vi "仪器参数改变发送 (子VI).vi"(8 "错误输入":errorcluster caption="错误输出") -> (0 "错误输出":errorcluster)   [LabVIEW 2016, in "数据传输系统-06.lvlib"]
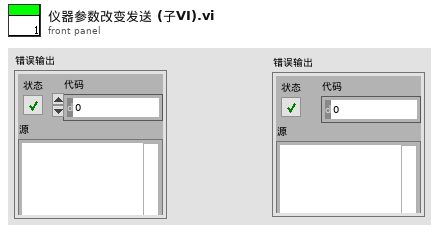
[diagram p1: front panel]
types:
  T1 = cluster{"测量量程":dbl, "测量精度":dbl, "测量间隔":dbl, "消解温度":dbl, "消解时长":dbl, "空白校准时间":timestamp, "曲线截距":dbl, "曲线斜率":dbl, "测量检出限":dbl, "测量信号值":dbl, "线性相关系数":dbl, "二次多项式系数":dbl, "标样校准时间":timestamp, "稀释倍数":dbl, "三项式系数":dbl, "空白标定系数":dbl, "量程系数":dbl, "F0/ORPA":dbl, "F1/ORPB":dbl, "F2/ORPK":dbl, "F3":dbl, "F4":dbl, "F5":dbl, "F6":dbl, "F7":dbl, "X0/滴定数":dbl, "量程":dbl}
  T2 = cluster{"CODMn关键参数":bool, "氨氮关键参数":bool, "总磷关键参数":bool, "总氮关键参数":bool, "CODCr关键参数":bool, "采配水关键参数":bool}
  T3 = cluster{"测量量程":dbl, "测量精度":dbl, "测量间隔":dbl, "消解温度":dbl, "消解时长":dbl, "空白校准时间":timestamp, "曲线截距":dbl, "曲线斜率":dbl, "测量检出限":dbl, "测量信号值":dbl, "线性相关系数":dbl, "二次多项式系数":dbl, "标样校准时间":timestamp, "稀释倍数":dbl, "三项式系数":dbl, "空白标定系数":dbl, "量程系数":dbl, "F0/ORPA":dbl, "F1/ORPB":dbl, "F2/ORPK":dbl, "F3":dbl, "F4":dbl, "F5":dbl, "F6":dbl, "F7":dbl, "X0/滴定数":dbl, "量程":dbl}[]
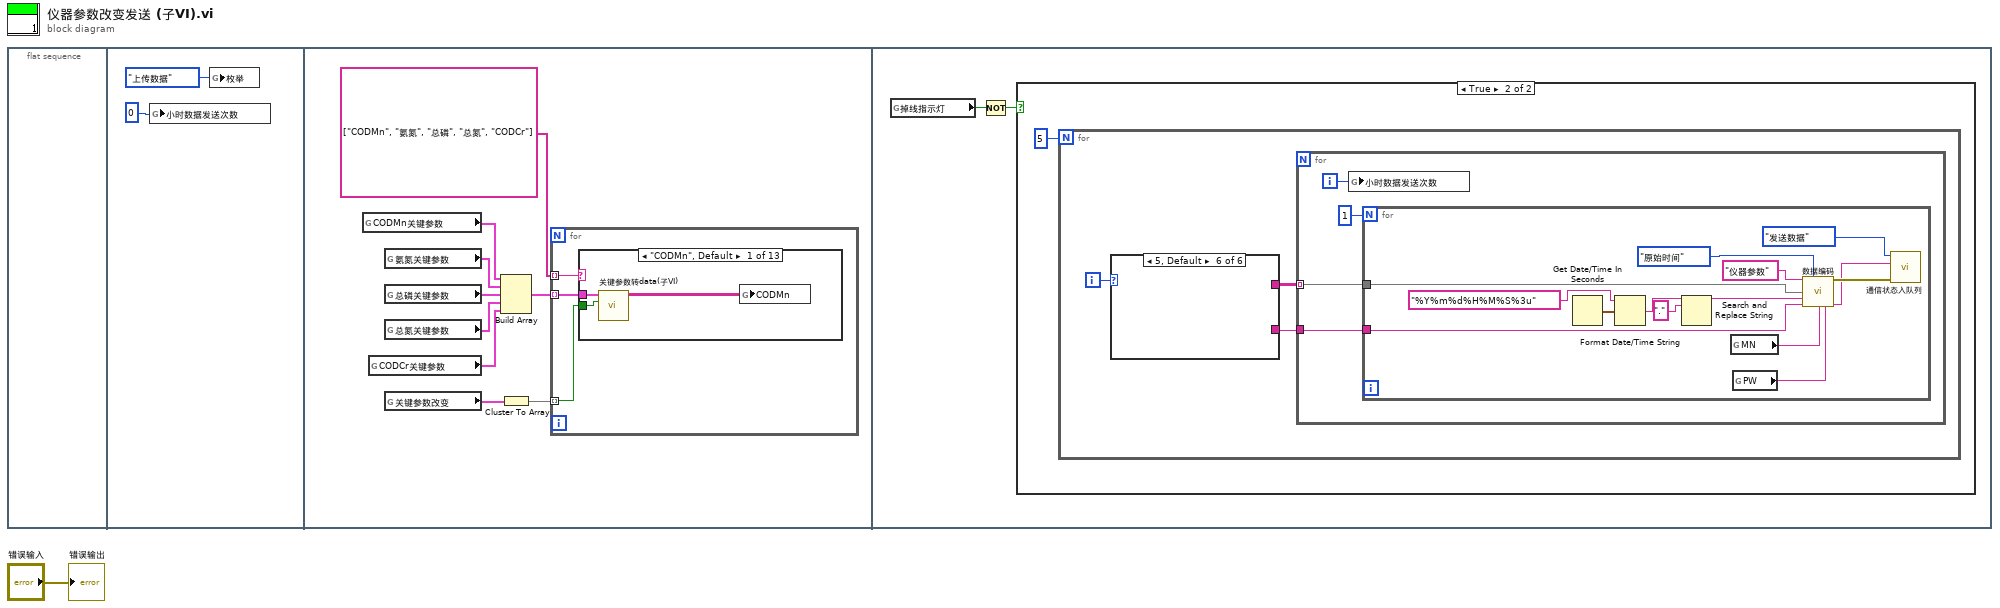
[diagram p0: block diagram]
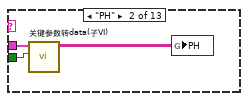
[diagram p2: hidden frame]
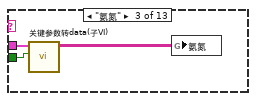
[diagram p3: hidden frame]
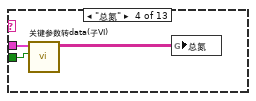
[diagram p4: hidden frame]
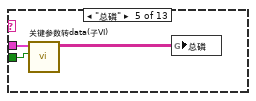
[diagram p5: hidden frame]
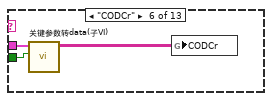
[diagram p6: hidden frame]
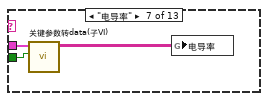
[diagram p7: hidden frame]
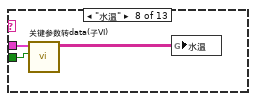
[diagram p8: hidden frame]
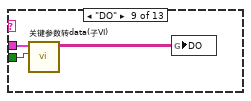
[diagram p9: hidden frame]
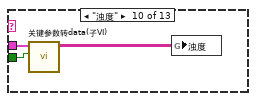
[diagram p10: hidden frame]
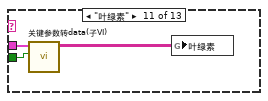
[diagram p11: hidden frame]
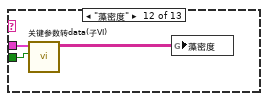
[diagram p12: hidden frame]
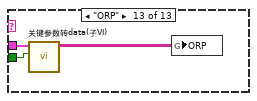
[diagram p13: hidden frame]
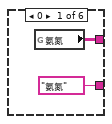
[diagram p15: hidden frame]
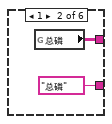
[diagram p16: hidden frame]
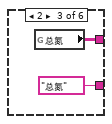
[diagram p17: hidden frame]
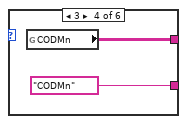
[diagram p18: hidden frame]
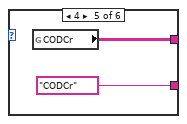
[diagram p19: hidden frame]
diagram:
  n1 = flat-sequence {
    frame #0 {
    }
    frame #1 {
      n2 = global write "全局 小时数据发送次数.vi" "小时数据发送次数"(0 ("小时数据发送次数")) -> ()
      n3 = global write "全局1.vi" "枚举"(enum16{"返回请求应答", "上传数据", "返回执行结果"}."上传数据" ("枚举")) -> ()
    }
    frame #2 {
      n4 = global read "全局1.vi" "CODMn关键参数"() -> (w9:T1)
      n5 = global read "全局1.vi" "CODCr关键参数"() -> (w12:T1)
      n6 = global read "全局1.vi" "氨氮关键参数"() -> (w11:T1)
      n7 = global read "全局1.vi" "总磷关键参数"() -> (w7:T1)
      n8 = global read "全局1.vi" "总氮关键参数"() -> (w6:T1)
      n9 = global read "全局1.vi" "关键参数改变"() -> (w5:T2)
      n10 = Build Array(w9, w11, w7, w6, w12) -> (w10:T3)
      n11 = Cluster To Array(cluster=w5) -> (array=w4:bool[])
      n12 = for {
        tunnel: string[] ["CODMn", "氨氮", "总磷", "总氮", "CODCr"] -> [w15] mode=indexing
        tunnel: w10 -> [w14] mode=indexing
        tunnel: w4 -> [w13] mode=indexing
        n13 = case shown="\"CODMn\", Default" w15 {
          tunnel: w14 -> [w17 w21 w24 w27 w30 w33 w36 w39 w42 w45 w48 w51 w54]
          tunnel: w13 -> [w16 w19 w22 w25 w28 w31 w34 w37 w40 w43 w46 w49 w52]
          frame "CODMn", Default {
            n14 = call "关键参数转data(子VI).vi"("改变?"=w16, "关键参数"=w17) -> ("数组"=w18:string[][])  [unwired: 9 in]
            n15 = global write "全局 所有参数.vi" "CODMn"(w18) -> ()
          }
          frame "PH" {
            n16 = call "关键参数转data(子VI).vi"("改变?"=w19, "关键参数"=w21) -> ("数组"=w20:string[][])  [unwired: 9 in]
            n17 = global write "全局 所有参数.vi" "PH"(w20) -> ()
          }
          frame "氨氮" {
            n18 = call "关键参数转data(子VI).vi"("改变?"=w22, "关键参数"=w24) -> ("数组"=w23:string[][])  [unwired: 9 in]
            n19 = global write "全局 所有参数.vi" "氨氮"(w23) -> ()
          }
          frame "总氮" {
            n20 = call "关键参数转data(子VI).vi"("改变?"=w25, "关键参数"=w27) -> ("数组"=w26:string[][])  [unwired: 9 in]
            n21 = global write "全局 所有参数.vi" "总氮"(w26) -> ()
          }
          frame "总磷" {
            n22 = call "关键参数转data(子VI).vi"("改变?"=w28, "关键参数"=w30) -> ("数组"=w29:string[][])  [unwired: 9 in]
            n23 = global write "全局 所有参数.vi" "总磷"(w29) -> ()
          }
          frame "CODCr" {
            n24 = call "关键参数转data(子VI).vi"("改变?"=w31, "关键参数"=w33) -> ("数组"=w32:string[][])  [unwired: 9 in]
            n25 = global write "全局 所有参数.vi" "CODCr"(w32) -> ()
          }
          frame "电导率" {
            n26 = call "关键参数转data(子VI).vi"("改变?"=w34, "关键参数"=w36) -> ("数组"=w35:string[][])  [unwired: 9 in]
            n27 = global write "全局 所有参数.vi" "电导率"(w35) -> ()
          }
          frame "水温" {
            n28 = call "关键参数转data(子VI).vi"("改变?"=w37, "关键参数"=w39) -> ("数组"=w38:string[][])  [unwired: 9 in]
            n29 = global write "全局 所有参数.vi" "水温"(w38) -> ()
          }
          frame "DO" {
            n30 = call "关键参数转data(子VI).vi"("改变?"=w40, "关键参数"=w42) -> ("数组"=w41:string[][])  [unwired: 9 in]
            n31 = global write "全局 所有参数.vi" "DO"(w41) -> ()
          }
          frame "浊度" {
            n32 = call "关键参数转data(子VI).vi"("改变?"=w43, "关键参数"=w45) -> ("数组"=w44:string[][])  [unwired: 9 in]
            n33 = global write "全局 所有参数.vi" "浊度"(w44) -> ()
          }
          frame "叶绿素" {
            n34 = call "关键参数转data(子VI).vi"("改变?"=w46, "关键参数"=w48) -> ("数组"=w47:string[][])  [unwired: 9 in]
            n35 = global write "全局 所有参数.vi" "叶绿素"(w47) -> ()
          }
          frame "藻密度" {
            n36 = call "关键参数转data(子VI).vi"("改变?"=w49, "关键参数"=w51) -> ("数组"=w50:string[][])  [unwired: 9 in]
            n37 = global write "全局 所有参数.vi" "藻密度"(w50) -> ()
          }
          frame "ORP" {
            n38 = call "关键参数转data(子VI).vi"("改变?"=w52, "关键参数"=w54) -> ("数组"=w53:string[][])  [unwired: 9 in]
            n39 = global write "全局 所有参数.vi" "ORP"(w53) -> ()
          }
        }
      }
    }
    frame #3 {
      n40 = global read "全局 数据发送重叠.vi" "掉线指示灯"() -> (w56:bool)
      n41 = Not(x=w56) -> (.not. x?=w55:bool)
      n42 = case shown="True" w55 {
        frame False {
        }
        frame True {
          n43 = for {
            N: 5 -> [_]
            i -> [w60]
            n44 = case shown="5, Default" w60 {
              tunnel: [w62 w64 w66 w68 w70 _] -> w59
              tunnel: ["氨氮" ("污染物编码") "总磷" ("污染物编码") "总氮" ("污染物编码") "CODMn" ("污染物编码") "CODCr" ("污染物编码") _] -> w58
              frame 0 {
                n45 = global read "全局 所有参数.vi" "氨氮"() -> (w62:string[][])
              }
              frame 1 {
                n46 = global read "全局 所有参数.vi" "总磷"() -> (w64:string[][])
              }
              frame 2 {
                n47 = global read "全局 所有参数.vi" "总氮"() -> (w66:string[][])
              }
              frame 3 {
                n48 = global read "全局 所有参数.vi" "CODMn"() -> (w68:string[][])
              }
              frame 4 {
                n49 = global read "全局 所有参数.vi" "CODCr"() -> (w70:string[][])
              }
              frame 5, Default {
              }
            }
            n50 = for {
              tunnel: w58 -> [w74]
              tunnel: w59 -> [w73] mode=indexing
              i -> [w72]
              n51 = global write "全局 小时数据发送次数.vi" "小时数据发送次数"(w72) -> ()
              n52 = for {
                N: 1 -> [_]
                tunnel: w74 -> [w79]
                tunnel: w73 -> [w78]
                n53 = Get Date/Time In Seconds() -> (seconds since 1Jan1904=w86:timestamp)
                n54 = Format Date/Time String(time format string (%c)="%Y%m%d%H%M%S%3u" ("时间格式字符串(%c)"), seconds (now)=w86) -> (date/time string=w85:string)  [unwired: 1 in]
                n55 = Search and Replace String(input string=w85, search string="." ("搜索字符串")) -> (result string=w83:string)  [unwired: 6 in, 3 out]
                n56 = global read "断电保存全局.vi" "MN"() -> (w82:string)
                n57 = global read "断电保存全局.vi" "PW"() -> (w81:string)
                n58 = call "数据编码.vi"("table输入"="仪器参数" ("新元素/子数组"), "仪器参数上传时间"=enum16{"精确到小时", "原始时间"}."原始时间", "仪器参数"=w78, "QN"=w83, "参数"=w79, "MN"=w82, "PW"=w81) -> ("错误常量"=w80:errorcluster, "通讯包字符串"=w75:string)  [unwired: 7 in]
                n59 = call "通信状态入队列.vi"("错误输入（无错误）"=w80, "发送报文"=w75, "枚举"=enum16{"打开连接", "发送数据", "读取数据", "数据处理", "关闭连接"}."发送数据") -> ()  [unwired: 8 in, 1 out]
              }
            }
          }
        }
      }
    }
  }
  "错误输出" <- "错误输入"
